vi "Create Comparison SubCluster.vi"(1 "Optimiser Cell in":refnum<class "Optimiser Cell.lvclass">) -> (0 "Cluster":T3 {"Observables"."Weight" min=0.0 max=1.0})   [LabVIEW 2020, in "Run Utilities.lvlib" / "Optimiser Cell.lvclass"]
doc: "Create a cluster of sorted data inside the class for comparing between two objects"
uses:
  Optimiser Cell.lvclass
  Optimisation observable.ctl
  Optimisation Strategy.ctl
  C:/LabVIEW Code/TALOS/talos/Run Utilities/Cell/Schedule Cell.lvclass
  9c8588eb-4ade-45cd-8c02-c3f35b0f03b2.vi
  5393bd10-604b-44c1-b98e-db4dae60dc14.vi
  4b3b17e5-a1d9-41d6-8b53-d92d233c5ecd.vi
  7cc20099-df9f-4d92-9d1c-6bd1f2c3a426.vi
  58772728-5576-494c-b300-3039281f2c0b.vi
  <vilib>/Comparison/Less/Less Functor/Less Functor.lvclass
  Optimiser Cell.lvclass/Optimiser Cell.ctl
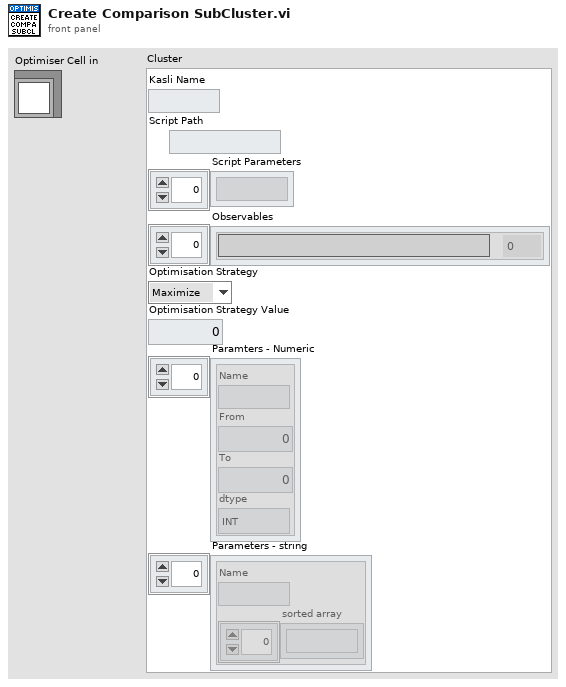
[diagram p1: front panel]
types:
  T1 = typedef "Run Utilities.lvlib/Optimiser Cell.lvclass/Optimisation observable.ctl" = cluster{"Name":string, "Weight":dbl}
  T2 = typedef "Run Utilities.lvlib/Optimiser Cell.lvclass/Optimisation Strategy.ctl" = enum16{"Maximize", "Minimize", "Value"}
  T3 = cluster{"Kasli Name":string, "Script Path":path, "Script Parameters":string[], "Observables":T1[], "Optimisation Strategy":T2, "Optimisation Strategy Value":dbl, "Paramters - Numeric":cluster{"Name":string, "From":dbl, "To":dbl, "dtype":enum16{"INT", "DBL"}}[], "Parameters - string":cluster{"Name":string, "sorted array":string[]}[]}
  T4 = typedef "Run Utilities.lvlib/Optimiser Cell.lvclass/Optimise parameter - numeric.ctl" = cluster{"Name":string, "Start value":dbl, "From":dbl, "To":dbl, "dtype":enum16{"INT", "DBL"}}
  T5 = typedef "Run Utilities.lvlib/Optimiser Cell.lvclass/Optimise parameter - string.ctl" = cluster{"Name":string, "Start value":string, "Options":string[]}
  T6 = cluster{"Name":string, "From":dbl, "To":dbl, "dtype":enum16{"INT", "DBL"}}
  T7 = cluster{"Name":string, "From":dbl, "To":dbl, "dtype":enum16{"INT", "DBL"}}[]
  T8 = cluster{"Name":string, "sorted array":string[]}[]
  T9 = cluster{"Accessors:FPGA Name":string, "Accessors:Script Path":path, "sorted array":string[], "sorted array":T1[], "Accessors:Optimisation Strategy":T2, "Accessors:Optimisation Strategy Value":dbl, "sorted array":cluster{"Name":string, "From":dbl, "To":dbl, "dtype":enum16{"INT", "DBL"}}[], "sorted array":cluster{"Name":string, "sorted array":string[]}[]}
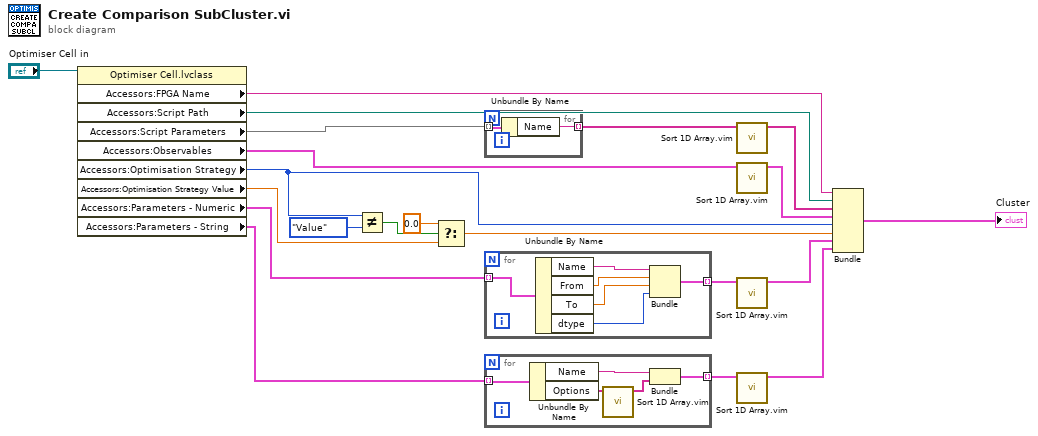
[diagram p0: block diagram]
diagram:
  n1 = property class="Optimiser Cell.lvclass"(reference="Optimiser Cell in") -> ("Accessors:FPGA Name"=w6:string, "Accessors:Script Path"=w7:path, "Accessors:Script Parameters"=w9:map{string, string}, "Accessors:Observables"=w8:T1[], "Accessors:Optimisation Strategy"=w13:T2, "Accessors:Optimisation Strategy Value"=w17:dbl, "Accessors:Parameters - Numeric"=w3:T4[], "Accessors:Parameters - String"=w2:T5[])  [unwired: 1 in, 2 out]
  n2 = Not Equal?(x=w13, y=Optimisation_Strategy."Value") -> (x != y?=w15:bool)
  n3 = Select(t=0.0, s=w15, f=w17) -> (s? t:f=w18:dbl)
  n4 = for {
    tunnel: w9 -> [w23] mode=indexing
    tunnel: [w22] -> w10 mode=indexing
    n5 = Unbundle By Name(w23) -> ("Name"=w22:string)
  }
  n6 = for {
    tunnel: w3 -> [w29] mode=indexing
    tunnel: [w27] -> w5 mode=indexing
    n7 = Unbundle By Name(w29) -> ("Name"=w28:string, "From"=w26:dbl, "To"=w25:dbl, "dtype"=w24:enum16{"INT", "DBL"})
    n8 = Bundle("Name"=w28, "From"=w26, "To"=w25, "dtype"=w24) -> (w27:T6)  [unwired: 1 in]
  }
  n9 = for {
    tunnel: w2 -> [w34] mode=indexing
    tunnel: [w30] -> w4 mode=indexing
    n10 = Unbundle By Name(w34) -> ("Name"=w33:string, "Options"=w32:string[])
    n11 = call "Sort 1D Array.vim"("unsorted array"=w32) -> ("sorted array"=w31:string[])  [unwired: 10 in]
    n12 = Bundle("Name"=w33, "sorted array"=w31) -> (w30:cluster{"Name":string, "sorted array":string[]})  [unwired: 1 in]
  }
  n13 = call "Sort 1D Array.vim"("unsorted array"=w10) -> ("sorted array"=w11:string[])  [unwired: 10 in]
  n14 = call "Sort 1D Array.vim"("unsorted array"=w8) -> ("sorted array"=w12:T1[])  [unwired: 10 in]
  n15 = call "Sort 1D Array.vim"("unsorted array"=w5) -> ("sorted array"=w19:T7)  [unwired: 10 in]
  n16 = call "Sort 1D Array.vim"("unsorted array"=w4) -> ("sorted array"=w20:T8)  [unwired: 10 in]
  n17 = Bundle("Accessors:FPGA Name"=w6, "Accessors:Script Path"=w7, "sorted array"=w11, "sorted array"=w12, "Accessors:Optimisation Strategy"=w13, "Accessors:Optimisation Strategy Value"=w18, "sorted array"=w19, "sorted array"=w20) -> (→"Cluster":T9)  [unwired: 1 in]
